vi "PI-TF_z.vi"(4 "reset-val":sgl format="%#_13g", 5 "u(k-1)":sgl format="%#_13g", 6 "reset":bool, 8 "Ki":sgl, 11 "e(k)":sgl format="%#_13g") -> (1 "u(k)":sgl)   [LabVIEW 2017]
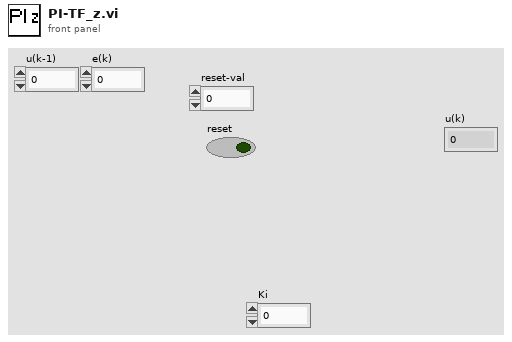
[diagram p1: front panel]
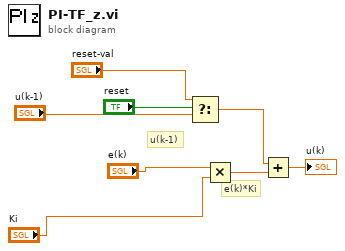
[diagram p0: block diagram]
diagram:
  # "e(k)*Ki"
  # "u(k-1)"
  n1 = Select(t="reset-val", s="reset", f="u(k-1)") -> (s? t:f=w5:sgl)
  n2 = Multiply(x="e(k)", y="Ki") -> (x*y=w8:sgl)
  n3 = Add(x=w5, y=w8) -> (x+y=→"u(k)":sgl)
